vi "OxITC503 _Config_ Program Complete Sweep.vi"(4 "error in (no error)":errorcluster, 6 "Sweep Program":T1(array[cluster]) {"Hold Time For Stage" min=0.0 max=1339.9 step=0.1 format="%.2f"; "Sweep Time for Stage" min=0.0 max=1339.9 step=0.1 format="%.2f"; "Set Point" format="%.2f"}, 7 "VISA session":refnum<visa-resource-name>) -> (0 "error out":errorcluster, 1 "VISA session":refnum<visa-resource-name>)   [LabVIEW 2013]
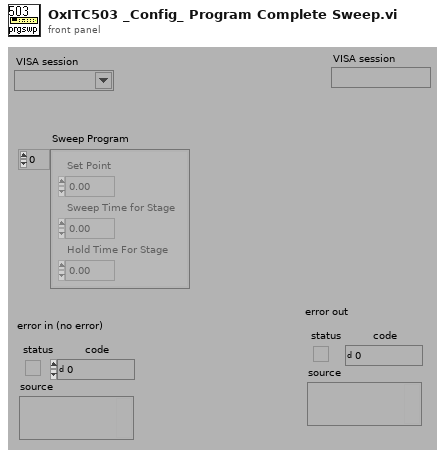
[diagram p1: front panel]
types:
  T1 = cluster{"Set Point":dbl, "Sweep Time for Stage":dbl, "Hold Time For Stage":dbl}[]
  T2 = enum16{"Local and locked", "Remote and Locked", "Local and unlocked", "Remote and Unlocked"}
  T3 = cluster{"System Status":i32, "Auto Status":enum16{"Heater and gas Manual", "Heater Auto, Gas Manual", "Heater Manual, Gas Auto", "Heater and Gas Auto"}, "Control Status":enum16{"Local and locked", "Remote and Locked", "Local and unlocked", "Remote and Unlocked"}, "Sweep Stage":i32, "Control Sensor":enum16{"Sensor 1", "Sensor 2", "Sensor 3"}, "Auto PID Status":enum16{"Auto PID Off", "Auto PID On"}}
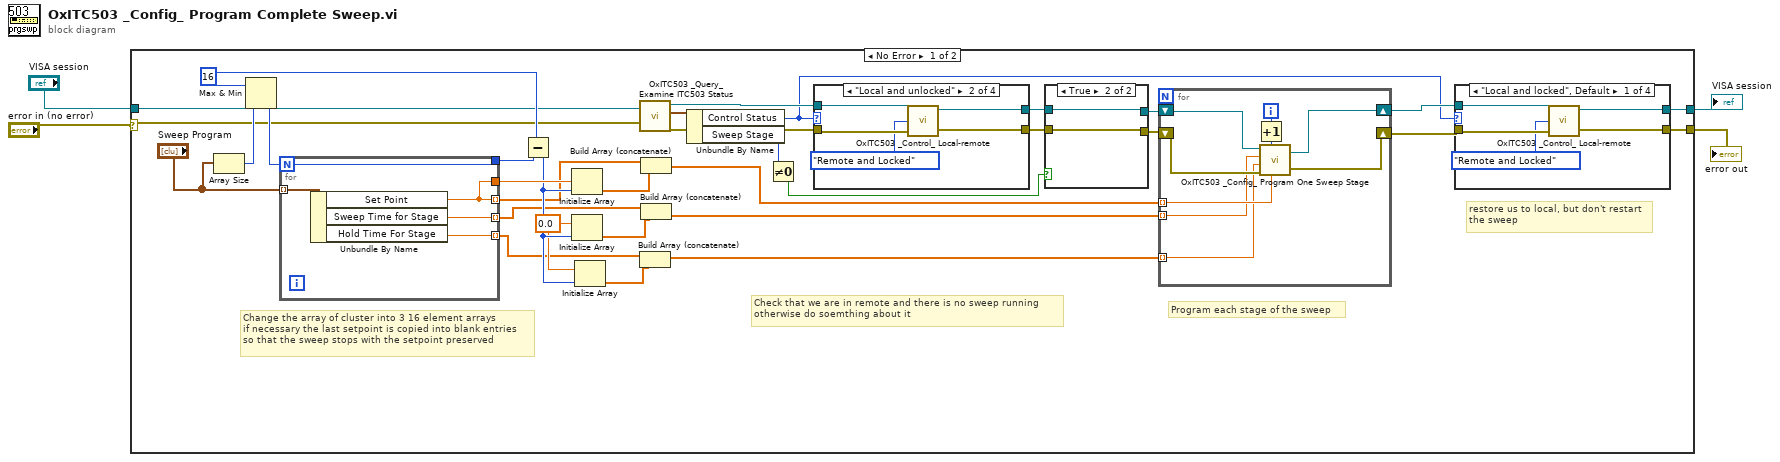
[diagram p0: block diagram]
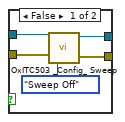
[diagram p2: hidden frame]
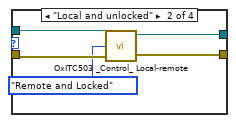
[diagram p3: hidden frame]
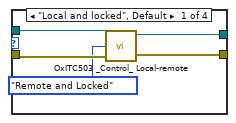
[diagram p6: hidden frame]
diagram:
  n1 = case shown="No Error" "error in (no error)" {
    selector: "error in (no error)" -> [w5 w87]
    tunnel: "VISA session" -> [w23 w88]
    tunnel: [w7 w87] -> w3
    tunnel: [w6 w88] -> w2
    frame No Error {
      w34 = 0.0 ("Element Data")
      w24 = 16 ("x")
      # "restore us to local, but don't restart\nthe sweep"
      # "Program each stage of the sweep"
      # "Check that we are in remote and there is no sweep running\notherwise do soemthing about it"
      # "Change the array of cluster into 3 16 element arrays\nif necessary the last setpoint is copied into blank entries\nso that the sweep stops with the setpoint preserved"
      n2 = Array Size(array="Sweep Program") -> (size(s)=w26:i32)
      n3 = Max & Min(x=w24, y=w26) -> (min(x,y)=w25:i32)  [unwired: 1 out]
      n4 = for {
        N: w25 -> [w86]
        tunnel: "Sweep Program" -> [w85] mode=indexing
        tunnel: [w86] -> w37
        tunnel: [w82] -> w28 mode=indexing
        tunnel: [w84] -> w29 mode=indexing
        tunnel: [w83] -> w30 mode=indexing
        tunnel: [w82] -> w36
        n5 = Unbundle By Name(w85) -> ("Set Point"=w82:dbl, "Sweep Time for Stage"=w84:dbl, "Hold Time For Stage"=w83:dbl)
      }
      n6 = Subtract(x=w24, y=w37) -> (x-y=w35:i32)
      n7 = Initialize Array(w36, w35) -> (w33:dbl[])
      n8 = Initialize Array(w34, w35) -> (w32:dbl[])
      n9 = Initialize Array(w34, w35) -> (w31:dbl[])
      n10 = call "OxITC503 _Query_ Examine ITC503 Status.vi"("VISA session"=w23, "error in"=w5) -> ("VISA session"=w21:refnum<visa-resource-name>, "ITC Status"=w22:T3, "error out (no error)"=w20:errorcluster)  [unwired: 1 out]
      n11 = Build Array (concatenate)(w30, w31) -> (w17:dbl[])
      n12 = Build Array (concatenate)(w28, w33) -> (w19:dbl[])
      n13 = Build Array (concatenate)(w29, w32) -> (w18:dbl[])
      n14 = Unbundle By Name(w22) -> ("Control Status"=w14:T2, "Sweep Stage"=w13:i32)
      n15 = Not Equal To 0?(x=w13) -> (x != 0?=w12:bool)
      n16 = case shown="\"Local and unlocked\"" w14 {
        tunnel: w21 -> [w72 w77 w79 w81]
        tunnel: w20 -> [w71 w76 w78 w80]
        tunnel: [w69 w74 w79 w81] -> w11
        tunnel: [w68 w73 w78 w80] -> w10
        frame "Local and locked", Default {
          n17 = call "OxITC503 _Control_ Local-remote.vi"("error in"=w71, "Control Status"=T2."Remote and Locked", "VISA session"=w72) -> ("error out (no error)"=w68:errorcluster, "VISA session"=w69:refnum<visa-resource-name>)
        }
        frame "Local and unlocked" {
          n18 = call "OxITC503 _Control_ Local-remote.vi"("error in"=w76, "Control Status"=T2."Remote and Locked", "VISA session"=w77) -> ("error out (no error)"=w73:errorcluster, "VISA session"=w74:refnum<visa-resource-name>)
        }
        frame "Remote and Locked" {
        }
        frame "Remote and Unlocked" {
        }
      }
      n19 = case shown="True" w12 {
        tunnel: w11 -> [w42 w44]
        tunnel: w10 -> [w41 w43]
        tunnel: [w39 w44] -> w9
        tunnel: [w38 w43] -> w8
        frame False {
          n20 = call "OxITC503 _Config_ Sweep.vi"("error in"=w41, "Sweep Status"=enum16{"Sweep Off", "Sweep On"}."Sweep Off", "VISA session"=w42) -> ("error out (no error)"=w38:errorcluster, "VISA session"=w39:refnum<visa-resource-name>)
        }
        frame True {
        }
      }
      n21 = for {
        shift-right: [w61] -> w16
        shift-left: w9 -> [w66]
        shift-right: [w60] -> w15
        shift-left: w8 -> [w65]
        tunnel: w19 -> [w64] mode=indexing
        tunnel: w18 -> [w63] mode=indexing
        tunnel: w17 -> [w62] mode=indexing
        i -> [w67]
        n22 = Increment(x=w67) -> (x+1=w59:i32)
        n23 = call "OxITC503 _Config_ Program One Sweep Stage.vi"("Setpoint for Stage"=w64, "Sweep Stage"=w59, "error in (no error)"=w65, "Hold Time For Stage"=w62, "Sweep Time for Stage"=w63, "VISA session"=w66) -> ("error out"=w60:errorcluster, "VISA session"=w61:refnum<visa-resource-name>)
      }
      n24 = case shown="\"Local and locked\", Default" w14 {
        tunnel: w16 -> [w49 w54 w56 w58]
        tunnel: w15 -> [w48 w53 w55 w57]
        tunnel: [w46 w51 w56 w58] -> w6
        tunnel: [w45 w50 w55 w57] -> w7
        frame "Local and locked", Default {
          n25 = call "OxITC503 _Control_ Local-remote.vi"("error in"=w48, "Control Status"=T2."Remote and Locked", "VISA session"=w49) -> ("error out (no error)"=w45:errorcluster, "VISA session"=w46:refnum<visa-resource-name>)
        }
        frame "Local and unlocked" {
          n26 = call "OxITC503 _Control_ Local-remote.vi"("error in"=w53, "Control Status"=T2."Remote and Locked", "VISA session"=w54) -> ("error out (no error)"=w50:errorcluster, "VISA session"=w51:refnum<visa-resource-name>)
        }
        frame "Remote and Locked" {
        }
        frame "Remote and Unlocked" {
        }
      }
    }
    frame Error {
    }
  }
  "VISA session" <- w2
  "error out" <- w3
